vi "DisConnectExit.vi"(7 "Event in":string, 10 "status":refnum<vi>, 11 "Ds PLCTags IN":T1[](array[typedef])) -> (2 "status？":bool, 3 "Event out":string)   [LabVIEW 2018]
uses:
  SubVIS.xio/DataSocket/DataSocket_Tags.ctl
  SubVIS.xio/DataSocket/Read PLC Vars/Read Bool Var.vi
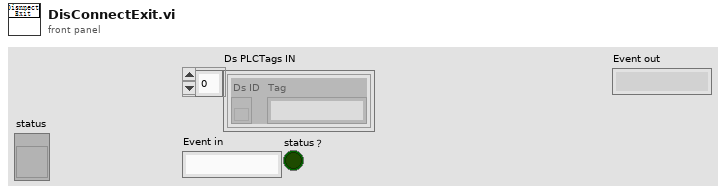
[diagram p1: front panel]
types:
  T1 = typedef "DataSocket_Tags.ctl" = cluster{"Ds ID":refnum<k13>, "Tag":string}
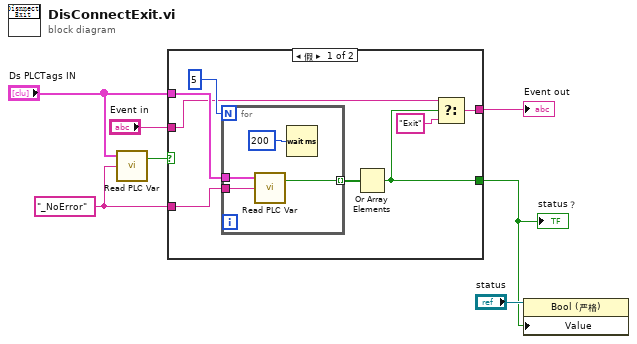
[diagram p0: block diagram]
diagram:
  w4 = "_NoError" ("Tag IN")
  n1 = call-poly "Read PLC Var.vi"("Tag IN"=w4, "Ds PLCTags IN"="Ds PLCTags IN") -> ("Bool Var out"=w7:bool)  [unwired: 1 in, 1 out]
  n2 = case shown="假" w7 {
    selector: w7 -> [_ w20]
    tunnel: "Event in" -> [w10 w21]
    tunnel: [w9 w21] -> w3
    tunnel: "Ds PLCTags IN" -> [w14 _]
    tunnel: w4 -> [w15 _]
    tunnel: [w8 w20] -> w1
    frame False {
      n3 = for {
        N: 5 -> [_]
        tunnel: w15 -> [w19]
        tunnel: w14 -> [w18]
        tunnel: [w16] -> w12 mode=indexing
        n4 = call-poly "Read PLC Var.vi"("Tag IN"=w19, "Ds PLCTags IN"=w18) -> ("Bool Var out"=w16:bool)  [unwired: 1 in, 1 out]
        n5 = Wait (ms)(milliseconds to wait=u32 200 ("等待时间（毫秒）")) -> ()  [unwired: 1 out]
      }
      n6 = Or Array Elements(Boolean array=w12) -> (logical OR=w8:bool)
      n7 = Select(t=w10, s=w8, f="Exit") -> (s? t:f=w9:string)
    }
    frame True {
    }
  }
  "Event out" <- w3
  "status？" <- w1
  n8 = property class="Bool (严格)"(reference="status", "Value"=w1) -> ()  [unwired: 1 in, 2 out]
